vi "C37 Get Analog Configuration.vi"(8 "error in (no error)":errorcluster, 9 "Analog Index":i32, 10 "PMU Index":i32, 11 "Pseudo PDC ID":i32) -> (0 "error out":errorcluster, 2 "Channel Name":string, 3 "Analog Configuration":T1)   [LabVIEW 2018, in "S3DK.lvlib" / "C37118-DLL.lvlib"]
uses:
  C37118-DLL.lvlib
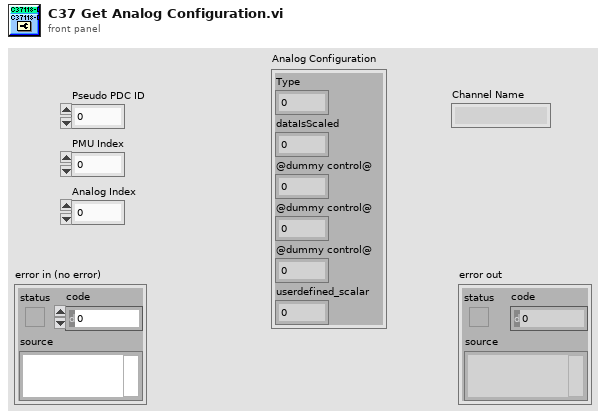
[diagram p1: front panel]
types:
  T1 = cluster{"Type":i32, "dataIsScaled":u8, "@dummy control@":i8, "@dummy control@":i8, "@dummy control@":i8, "userdefined_scalar":sgl}
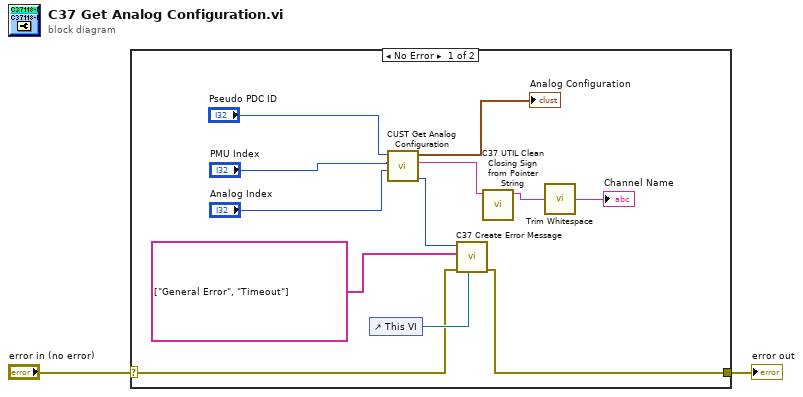
[diagram p0: block diagram]
diagram:
  n1 = case shown="No Error" "error in (no error)" {
    selector: "error in (no error)" -> [w13 w15]
    tunnel: [w12 w15] -> w2
    frame No Error {
      n2 = control-ref of="This VI"() -> (w14:refnum<vi>)
      n3 = call "CUST Get Analog Configuration.vi"("analogIndex"="Analog Index", "pmuIndex"="PMU Index", "pseudoPdcId"="Pseudo PDC ID") -> ("function return"=w3:i32, "name out"=w4:string, "analogCfg out"=→"Analog Configuration":T1)  [unwired: 6 in]
      n4 = call "C37 Create Error Message.vi"("VI Reference"=w14, "error in (no error)"=w13, "Error Messages"=string[] ["General Error", "Timeout"], "function return"=w3) -> ("error out"=w12:errorcluster)  [unwired: 7 in]
      n5 = call "C37 UTIL Clean Closing Sign from Pointer String.vi"("String In"=w4) -> ("String Out"=w9:string)  [unwired: 10 in]
      n6 = call <vilib>:"Trim Whitespace.vi"("string"=w9) -> ("trimmed string"=→"Channel Name":string)  [unwired: 1 in]
    }
    frame Error {
    }
  }
  "error out" <- w2
